vi "Get Parameter Value (JSON).vi"(10 "Parameter Name":string, 11 "JSON":string) -> (1 "Found":bool, 2 "Parameter Value":string, 3 "Remaining JSON":string, 4 "Null":bool)   [LabVIEW 2015, in "NI_Azure_JSON Parsing.lvlib"]
uses:
  NI_Azure_JSON Parsing.lvlib
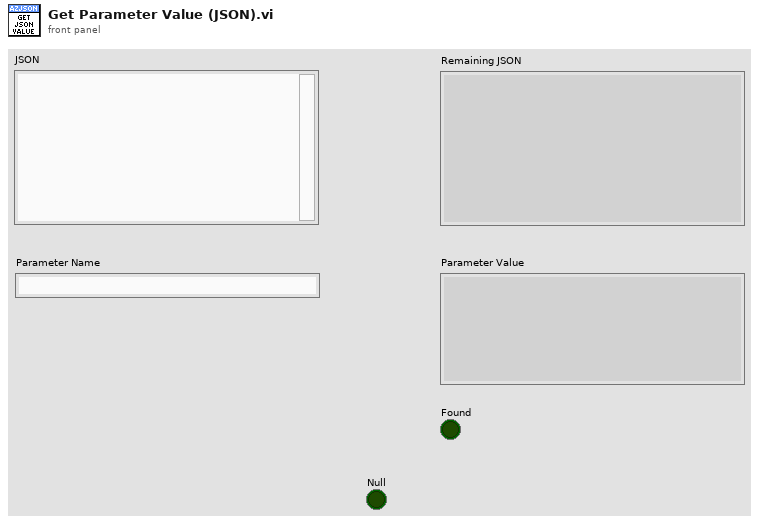
[diagram p1: front panel]
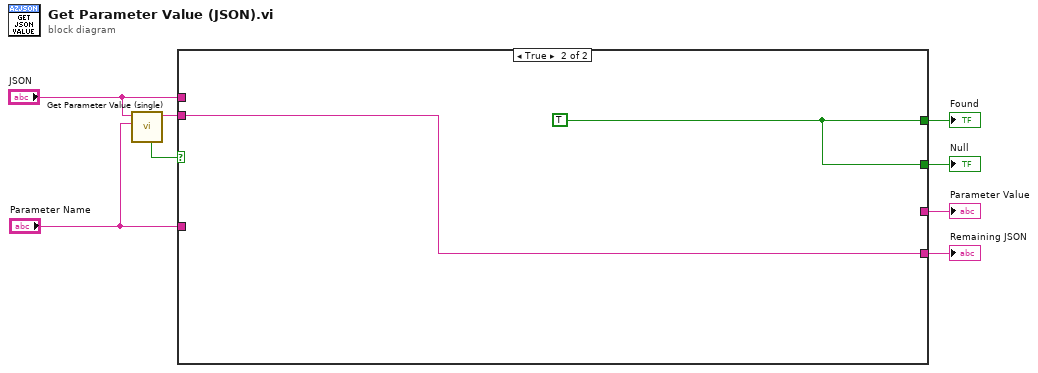
[diagram p0: block diagram]
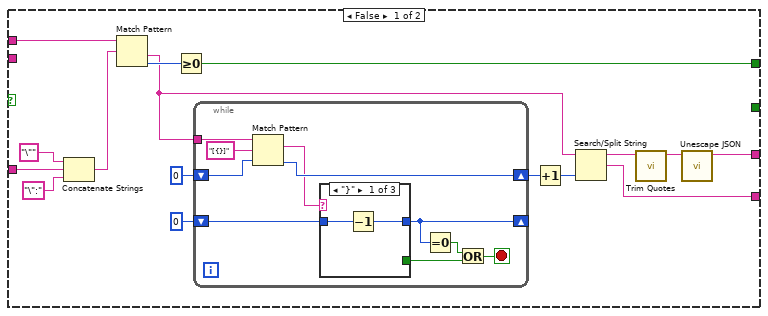
[diagram p2: hidden frame]
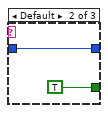
[diagram p3: hidden frame]
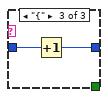
[diagram p4: hidden frame]
diagram:
  n1 = call "Get Parameter Value (single).vi"("Parameter Name"="Parameter Name", "JSON"="JSON") -> ("Remaining JSON"=w2:string, "Null"=w3:bool)  [unwired: 6 in, 2 out]
  n2 = case shown="True" w3 {
    tunnel: [w20 w41] -> w8
    tunnel: [w15 w42] -> w7
    tunnel: [w11 _] -> w6
    tunnel: "JSON" -> [w10 _]
    tunnel: "Parameter Name" -> [w9 _]
    tunnel: w2 -> [_ w42]
    tunnel: [_ w41] -> w1
    frame False {
      n3 = Concatenate Strings("\"" ("string"), w9, "\":" ("string")) -> (w24:string)
      n4 = Match Pattern(string=w10, regular expression=w24) -> (after substring=w16:string, offset past match=w21:i32)  [unwired: 1 in, 2 out]
      n5 = Greater Or Equal To 0?(x=w21) -> (x >= 0?=w20:bool)
      n6 = while {
        tunnel: w16 -> [w32]
        shift-right: [w31] -> w17
        shift-left: 0 -> [w33]
        shift-right: [w28] -> _
        shift-left: 0 -> [w30]
        stop <- w25 stop-if-true
        n7 = Match Pattern(string=w32, regular expression="[{}]", offset (0)=w33) -> (match substring=w29:string, offset past match=w31:i32)  [unwired: 2 out]
        n8 = case shown="\"}\"" w29 {
          tunnel: w30 -> [w36 w37 w40]
          tunnel: [_ TRUE _] -> w27
          tunnel: [w35 w37 w39] -> w28
          frame "}" {
            n9 = Decrement(x=w36) -> (x-1=w35:i32)
          }
          frame Default {
          }
          frame "{" {
            n10 = Increment(x=w40) -> (x+1=w39:i32)
          }
        }
        n11 = Equal To 0?(x=w28) -> (x = 0?=w26:bool)
        n12 = Or(x=w26, y=w27) -> (x .or. y?=w25:bool)
      }
      n13 = Increment(x=w17) -> (x+1=w14:i32)
      n14 = Search/Split String(string=w16, offset (0)=w14) -> (substring before match=w13:string, match + rest of string=w15:string)  [unwired: 1 in, 1 out]
      n15 = call "Trim Quotes.vi"("String"=w13) -> ("String without Quotes"=w12:string)  [unwired: 9 in, 1 out]
      n16 = call "Unescape JSON.vi"("Escaped JSON"=w12) -> ("Unescaped JSON"=w11:string)  [unwired: 10 in]
    }
    frame True {
      w41 = TRUE
    }
  }
  "Parameter Value" <- w6
  "Remaining JSON" <- w7
  "Found" <- w8
  "Null" <- w1
